vi "ErrorCheckHWI.vi"(8 "error in (no error)":errorcluster, 11 "Slave_Pulseblaster in":refnum<class "Slave_Pulseblaster.lvclass">) -> (0 "error out":errorcluster, 3 "Slave_Pulseblaster out":refnum<class "Slave_Pulseblaster.lvclass">)   [LabVIEW 2013, in "Slave_Pulseblaster.lvclass"]
uses:
  Slave_Pulseblaster.lvclass
  Device/Device.lvclass
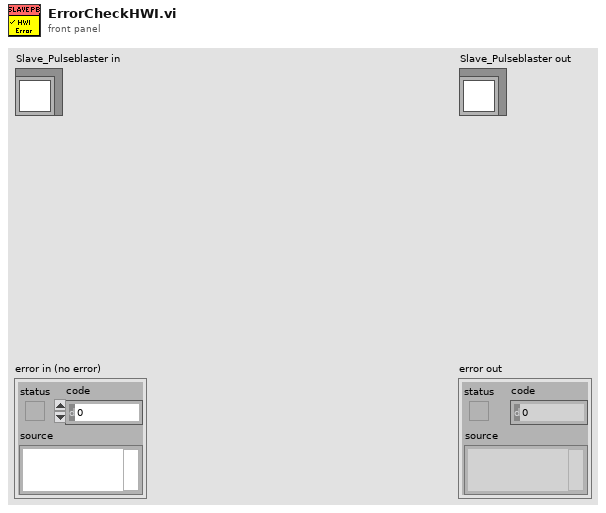
[diagram p1: front panel]
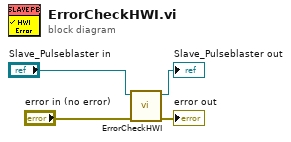
[diagram p0: block diagram]
diagram:
  n1 = call-parent "ErrorCheckHWI.vi"("error in (no error)"="error in (no error)", "Device in"="Slave_Pulseblaster in") -> ("error out"=→"error out":errorcluster, "Device out"=→"Slave_Pulseblaster out":refnum<class "Slave_Pulseblaster.lvclass">)  [unwired: 8 in]
